vi "SH_readShapelets.vi"(8 "error in":errorcluster, 11 "Shapelets File":path) -> (0 "error out":errorcluster, 1 "Array of Shapelets":cluster{dbl[][]}[](array[cluster]), 2 "size(s)":i32[](array[numeric]))   [LabVIEW 2016, in "Shapelets Search (Brute Force).lvlib"]
uses:
  Shapelets Search (Brute Force).lvlib
panel:
  # "This VI is a part of BCI Design library, http://www.ru-bci.org \nCopyright © 2020, Sotnikov Peter, All rights reserved. License: GNU GPLv3"
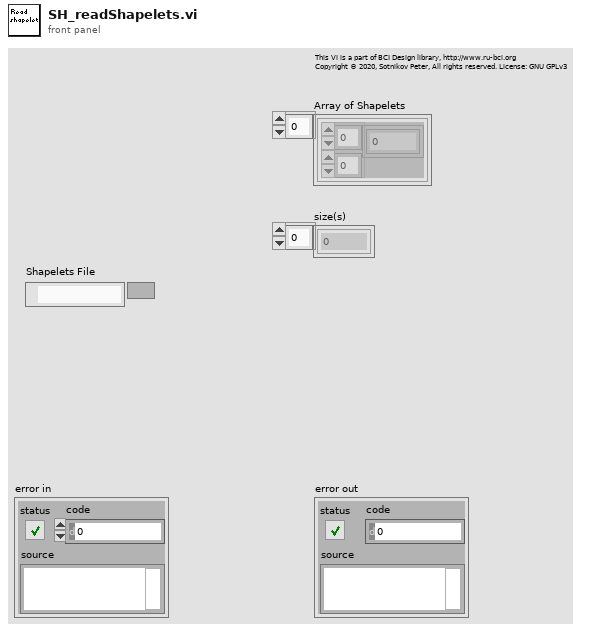
[diagram p1: front panel]
types:
  T1 = enum16{"big-endian, network order", "native, host order", "little-endian"}
  T2 = enum16{"open", "replace", "create", "open or create", "replace or create", "replace or create with confirmation"}
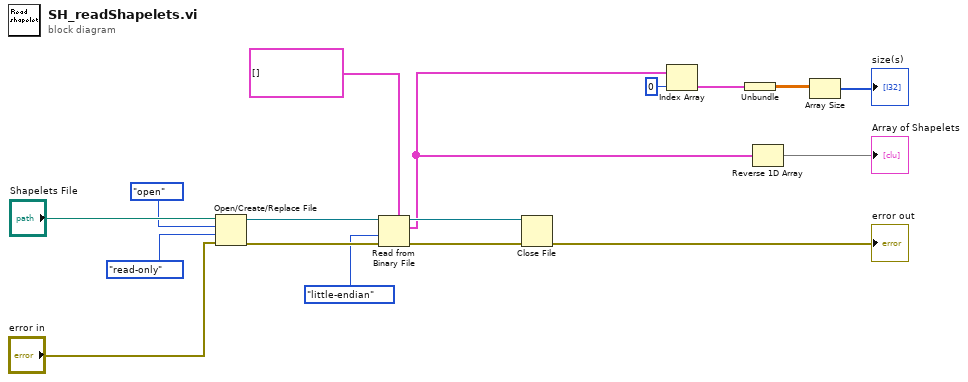
[diagram p0: block diagram]
diagram:
  n1 = Open/Create/Replace File(file path (use dialog)="Shapelets File", error in="error in", operation (0:open)=T2."open", access (0:read/write)=enum16{"read/write", "read-only", "write-only"}."read-only") -> (refnum out=w13:refnum<file>, error out=w12:errorcluster)  [unwired: 2 in, 1 out]
  n2 = Read from Binary File(5:cluster{dbl[][]}[] [] ("Array of Shapelets"), 8:w12, 9:T1."little-endian" ("byte order (0:big-endian, network order)"), 11:w13) -> (0:w9:errorcluster, 2:w2:cluster{dbl[][]}[], 3:w10:refnum<file>)  [unwired: 2 in, 1 out]
  n3 = Close File(refnum=w10, error in=w9) -> (error out=→"error out":errorcluster)  [unwired: 1 out]
  n4 = Index Array(array=w2, index=0) -> (element=w5:cluster{dbl[][]})
  n5 = Unbundle(w5) -> (w4:dbl[][])
  n6 = Reverse 1D Array(array=w2) -> (reversed array=→"Array of Shapelets":cluster{dbl[][]}[])
  n7 = Array Size(array=w4) -> (size(s)=→"size(s)":i32[])
